vi "Metronome.vi"(5 "initialize":bool, 7 "start time (ns)":u64, 9 "loop period (ns)":u32=500) -> (1 "time snapped event":bool, 3 "finished late?":bool)   [LabVIEW 2015, in "FPGA Timekeeper.lvlib"]
doc: "Synchronizes execution rate of a loop."
uses:
  FPGA Timekeeper.lvlib
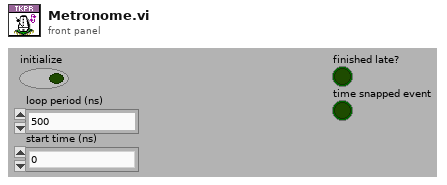
[diagram p1: front panel]
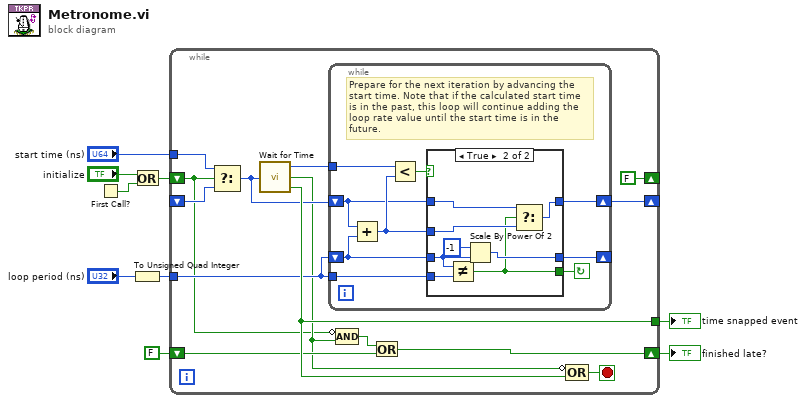
[diagram p0: block diagram]
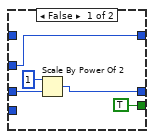
[diagram p2: hidden frame]
diagram:
  n1 = First Call?() -> (First Call?: T/F=w8:bool)
  n2 = To Unsigned Quad Integer(1:"loop period (ns)") -> (0:w2:u64)
  n3 = Or(x="initialize", y=w8) -> (x .or. y?=w6:bool)
  n4 = while {
    shift-right: [w23] -> w3
    shift-left: FALSE ("Time already elapsed") -> [w19]
    tunnel: [w21] -> w4
    shift-right: [FALSE] -> _
    shift-left: w6 -> [w10]
    shift-right: [w17] -> _
    shift-left: _ -> [w15]
    tunnel: w2 -> [w16]
    tunnel: "start time (ns)" -> [w13]
    stop <- w22 stop-if-true
    n5 = Select(t=w13, s=w10, f=w15) -> (s? t:f=w14:u64)
    n6 = call "Wait for Time.vi"("future time (ns)"=w14) -> ("time snapped event"=w21:bool, "time already elapsed"=w11:bool, "return time (ns)"=w18:u64)
    n7 = while {
      tunnel: w18 -> [w31]
      shift-right: [w25] -> w17
      shift-left: w14 -> [w24]
      tunnel: w16 -> [w29]
      shift-right: [w27] -> _
      shift-left: w16 -> [w30]
      stop <- w28 continue-if-true
      # "Prepare for the next iteration by advancing the start time. Note that if the calculated start time is in the past, this loop will continue adding the loop rate value until the start time is in the future."
      n8 = Add(x=w24, y=w30) -> (x+y=w26:u64)
      n9 = Less?(x=w31, y=w26) -> (x < y?=w32:bool)
      n10 = case shown="True" w32 {
        tunnel: w30 -> [w37 w44]
        tunnel: w29 -> [_ w45]
        tunnel: [TRUE w38] -> w28
        tunnel: [w36 w42] -> w27
        tunnel: w26 -> [w33 w41]
        tunnel: [w33 w39] -> w25
        tunnel: w24 -> [_ w40]
        frame False {
          n11 = Scale By Power Of 2(n=1, x=w37) -> (x*2^n=w36:u64)
        }
        frame True {
          n12 = Not Equal?(x=w44, y=w45) -> (x != y?=w38:bool)
          n13 = Scale By Power Of 2(n=-1, x=w44) -> (x*2^n=w42:u64)
          n14 = Select(t=w40, s=w38, f=w41) -> (s? t:f=w39:u64)
        }
      }
    }
    n15 = Compound Arithmetic op=AND(invert w10, w11) -> (w12:bool)
    n16 = Or(x=w12, y=w19) -> (x .or. y?=w23:bool)
    n17 = Compound Arithmetic op=OR(invert w11, w21) -> (w22:bool)
  }
  "finished late?" <- w3
  "time snapped event" <- w4
